vi "Update HW Configuration File Dependency.vi"(8 "error in (no error)":errorcluster, 10 "Node Ptr dup":T1 format="%.0x", 11 "selected path in":path) -> (0 "error out":errorcluster)   [LabVIEW 2016, in "Ballard Arinc-429 System Explorer.lvlib"]
uses:
  Ballard Arinc-429 System Explorer.lvlib
  <vilib>/NI Veristand/Custom Device API/Custom Device Item Ref.ctl
  <vilib>/NI Veristand/Custom Device API/Custom Device File Dependency.ctl
  <vilib>/NI Veristand/Custom Device API/Path Specification.ctl
  <vilib>/NI Veristand/Custom Device API/Path Type.ctl
  <vilib>/NI Veristand/Custom Device API/Custom Device Supported Target.ctl
  Shared/Controls and Global/Initialization Method.ctl
  Shared/Controls and Global/Global.vi
  <vilib>/NI Veristand/Custom Device API/Get Item Property (I32).vi
  <vilib>/NI Veristand/Custom Device API/Get Item Property (U16).vi
  <vilib>/NI VeriStand/Custom Device API/Custom Device API.lvlib
  Shared/Ballard Arinc-429 Shared.lvlib
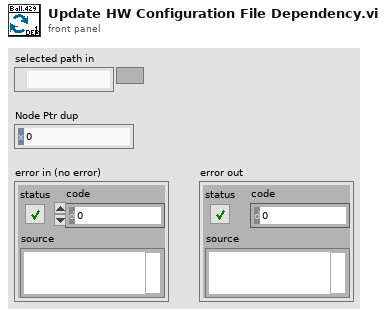
[diagram p1: front panel]
types:
  T1 = typedef "Custom Device API.lvlib/Custom Device Item Ref.ctl" = u64
  T2 = typedef "Ballard Arinc-429 Shared.lvlib/Initialization Method.ctl" = enum16{"PXI Slot Number", "Card Number"}
  T3 = typedef "Custom Device API.lvlib/Custom Device Supported Target.ctl" = enum16{"All", "PharLap", "VxWorks", "Windows", "Linux_32_ARM", "Linux_x64", "PharLap & Windows", "PharLap & VxWorks", "VxWorks & Windows"}
  T4 = typedef "Custom Device API.lvlib/Custom Device File Dependency.ctl" = cluster{"Source":T5, "RT Destination":path, "ForceDownload?":bool, "SupportedTarget":T3, "Version":string}
  T5 = typedef "Custom Device API.lvlib/Path Specification.ctl" = cluster{"Path":path, "Type":T6}
  T6 = typedef "Custom Device API.lvlib/Path Type.ctl" = enum16{"Absolute", "To Base", "To Common Data Dir", "To Application Data Dir"}
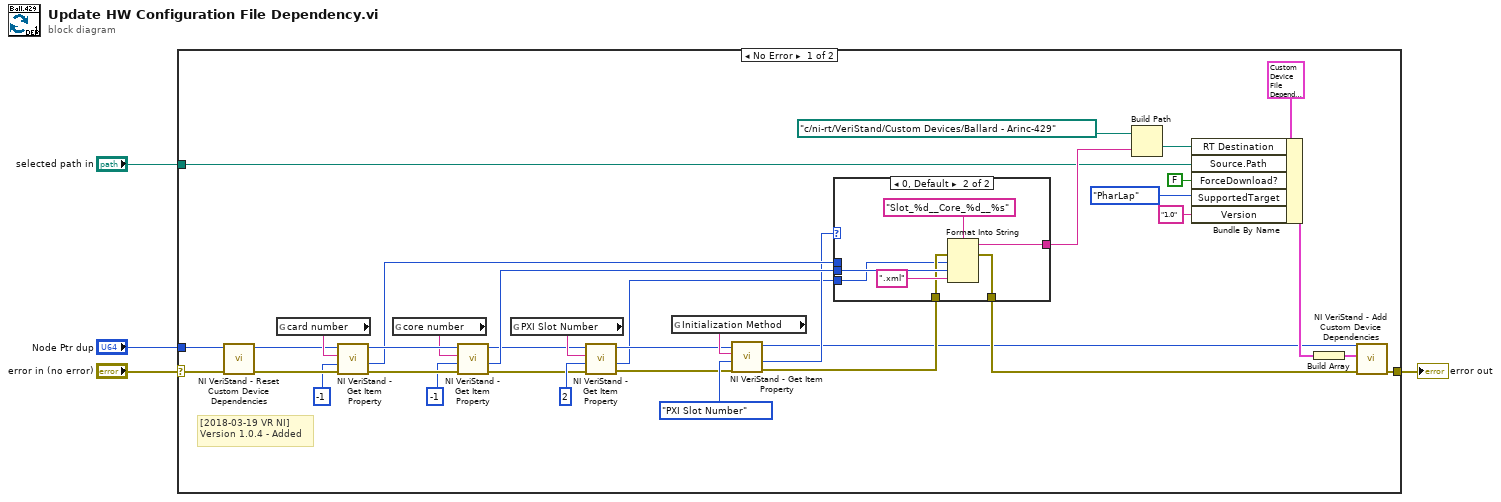
[diagram p0: block diagram]
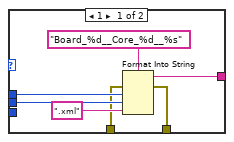
[diagram p2: hidden frame]
diagram:
  n1 = case shown="No Error" "error in (no error)" {
    selector: "error in (no error)" -> [w31 w55]
    tunnel: "Node Ptr dup" -> [w40 _]
    tunnel: "selected path in" -> [w5 _]
    tunnel: [w38 w55] -> w2
    frame No Error {
      # "[2018-03-19 VR NI]\nVersion 1.0.4 - Added"
      n2 = call <vilib>:"NI VeriStand - Reset Custom Device Dependencies.vi"("error in (no error)"=w31, "Device Ref in"=w40) -> ("error out"=w26:errorcluster, "Device Ref out"=w27:T1)  [unwired: 8 in]
      n3 = global read "Global.vi" "card number"() -> (w30:string)
      n4 = call-poly <vilib>:"NI VeriStand - Get Item Property.vi"("error in (no error)"=w26, "Default Value"=-1, "Property Name"=w30, "Item Ref in"=w27) -> ("error out"=w29:errorcluster, "Value"=w24:i32, "Item Ref out"=w28:T1)  [unwired: 4 in, 1 out]
      n5 = global read "Global.vi" "core number"() -> (w25:string)
      n6 = call-poly <vilib>:"NI VeriStand - Get Item Property.vi"("error in (no error)"=w29, "Default Value"=-1, "Property Name"=w25, "Item Ref in"=w28) -> ("error out"=w11:errorcluster, "Value"=w23:i32, "Item Ref out"=w12:T1)  [unwired: 4 in, 1 out]
      n7 = global read "Global.vi" "PXI Slot Number"() -> (w14:string)
      n8 = call-poly <vilib>:"NI VeriStand - Get Item Property.vi"("error in (no error)"=w11, "Default Value"=2, "Property Name"=w14, "Item Ref in"=w12) -> ("error out"=w10:errorcluster, "Value"=w7:i32, "Item Ref out"=w9:T1)  [unwired: 4 in, 1 out]
      n9 = global read "Global.vi" "Initialization Method"() -> (w18:string)
      n10 = call-poly <vilib>:"NI VeriStand - Get Item Property.vi"("error in (no error)"=w10, "Default Value"=Initialization_Method."PXI Slot Number" ("Initialization Method"), "Property Name"=w18, "Item Ref in"=w9) -> ("error out"=w17:errorcluster, "Value"=w15:u16, "Item Ref out"=w8:T1)  [unwired: 4 in, 1 out]
      n11 = case shown="0, Default" w15 {
        tunnel: w24 -> [w47 _]
        tunnel: w23 -> [w46 w54]
        tunnel: [w45 w53] -> w22
        tunnel: [w44 w52] -> w21
        tunnel: w17 -> [w41 w49]
        tunnel: w7 -> [_ w48]
        frame 1 {
          n12 = Format Into String(format string="Board_%d__Core_%d__%s", error in=w41, w47, w46, ".xml" ("input 3")) -> (resulting string=w45:string, error out=w44:errorcluster)  [unwired: 1 in]
        }
        frame 0, Default {
          n13 = Format Into String(format string="Slot_%d__Core_%d__%s", error in=w49, w48, w54, ".xml" ("input 3")) -> (resulting string=w53:string, error out=w52:errorcluster)  [unwired: 1 in]
        }
      }
      n14 = Build Path(base path=path "c:/ni-rt/VeriStand/Custom Devices/Ballard - Arinc-429" ("RT Destination"), name or relative path=w22) -> (appended path=w6:path)
      n15 = Bundle By Name(cluster=T4 {"Source"={"Path"=path "", "Type"=enum."Absolute"}, "RT Destination"=path "", "ForceDownload?"=FALSE, "SupportedTarget"=enum."PharLap", "Version"=""} ("Dependency"), "RT Destination"=w6, "Source.Path"=w5, "ForceDownload?"=FALSE, "SupportedTarget"=Custom_Device_Supported_Target."PharLap", "Version"="1.0") -> (w32:T4)
      n16 = Build Array(w32) -> (w33:T4[])
      n17 = call <vilib>:"NI VeriStand - Add Custom Device Dependencies.vi"("error in (no error)"=w21, "Dependencies"=w33, "Device Ref in"=w8) -> ("error out"=w38:errorcluster)  [unwired: 7 in, 1 out]
    }
    frame Error {
    }
  }
  "error out" <- w2
